vi "Motor R Control.vi"(1 "Motor Axis Pos":i32, 2 "Game Axis Pos":i32) -> (0 "Motor Move":string)   [LabVIEW 2013]
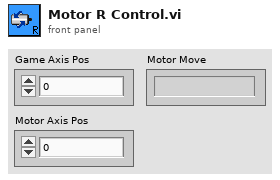
[diagram p1: front panel]
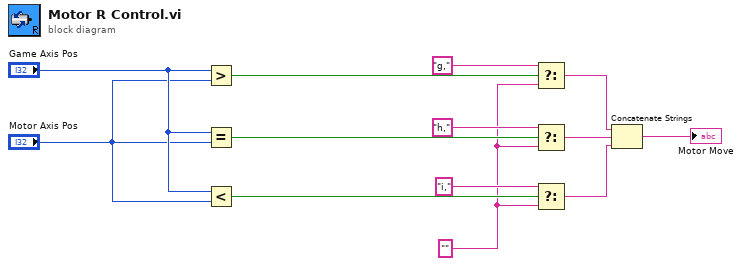
[diagram p0: block diagram]
diagram:
  w2 = ""
  n1 = Greater?(x="Game Axis Pos", y="Motor Axis Pos") -> (0:w11:bool)
  n2 = Equal?(x="Game Axis Pos", y="Motor Axis Pos") -> (x = y?=w10:bool)
  n3 = Less?(x="Game Axis Pos", y="Motor Axis Pos") -> (x < y?=w9:bool)
  n4 = Select(t="g,", s=w11, f=w2) -> (s? t:f=w3:string)
  n5 = Select(t="h,", s=w10, f=w2) -> (s? t:f=w5:string)
  n6 = Select(t="i,", s=w9, f=w2) -> (s? t:f=w4:string)
  n7 = Concatenate Strings(w3, w5, w4) -> (→"Motor Move":string)
